vi "CreateLicenseKeyPC.vi"(8 "error in":errorcluster, 10 "Serial number":string, 11 "IP address (localhost)":string="169.254.1.19") -> (0 "error out":errorcluster)   [LabVIEW 2020]
uses:
  <vilib>/Utility/config.llb/Write Key (String).vi
  <vilib>/WebDAVClient/Advanced/Put File.vi
  <vilib>/Utility/config.llb/NI_LVConfig.lvlib
  <vilib>/WebDAVClient/NI_WebDAV.lvlib
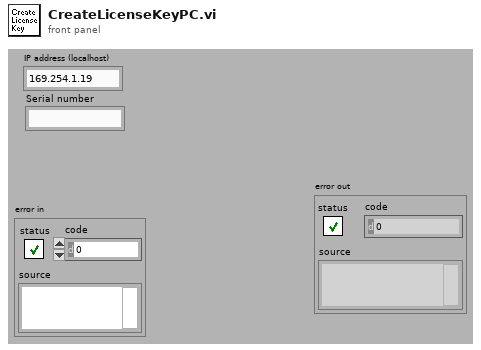
[diagram p1: front panel]
types:
  T1 = typedef "NI_LVConfig.lvlib/Config Data RefNum.ctl" = refnum<k1>
  T2 = typedef "NI_WebDAV.lvlib/SessionHandle.ctl" = refnum<k1>
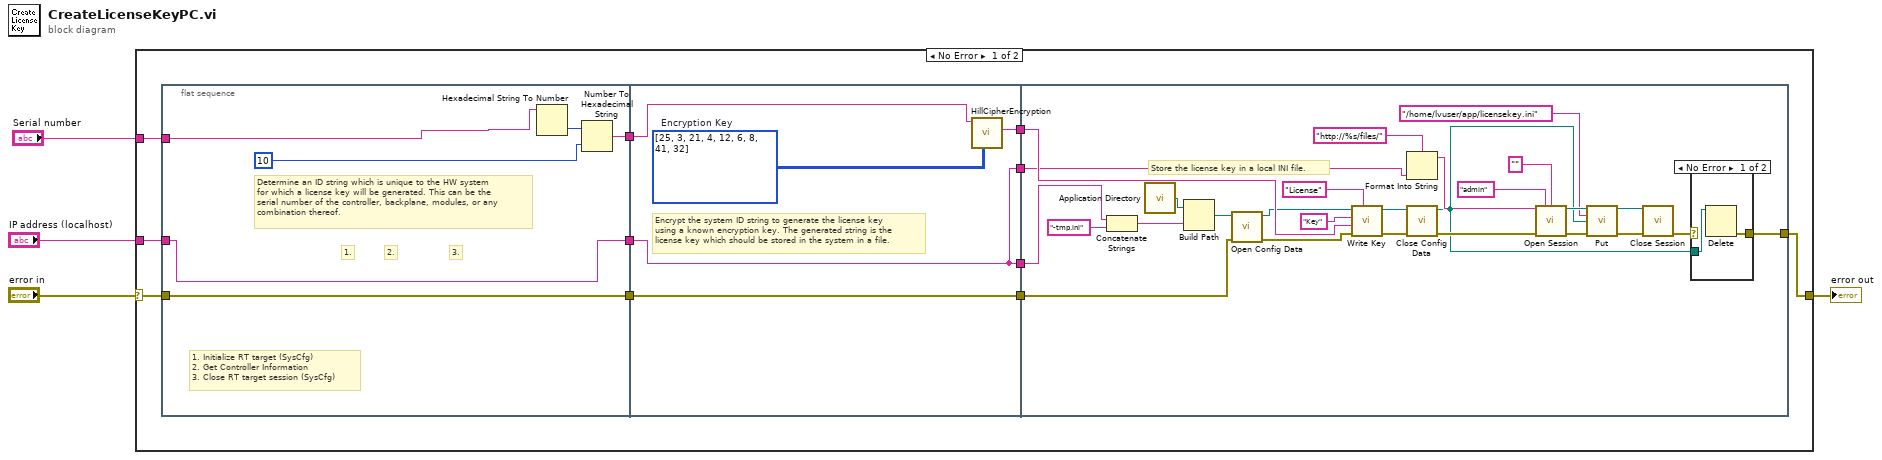
[diagram p0: block diagram]
diagram:
  n1 = case shown="No Error" "error in" {
    selector: "error in" -> [w7 w57]
    tunnel: "IP address (localhost)" -> [w8 _]
    tunnel: [w6 w57] -> w2
    tunnel: "Serial number" -> [w5 _]
    frame No Error {
      n2 = flat-sequence {
        tunnel: [w20] -> w15
        tunnel: [w17] -> w14
        tunnel: w8 -> [w18]
        tunnel: [w18] -> w13
        tunnel: w7 -> [w17]
        tunnel: w5 -> [w16]
        tunnel: w15 -> [w25]
        tunnel: [w24] -> w12
        tunnel: [w23] -> w11
        tunnel: w14 -> [w23]
        tunnel: [w22] -> w10
        tunnel: w13 -> [w22]
        tunnel: [w22] -> w9
        tunnel: w12 -> [w53]
        tunnel: w11 -> [w41]
        tunnel: w10 -> [w46]
        tunnel: w9 -> [w39]
        tunnel: [w28] -> w6
        frame #0 {
          # "3."
          # "2."
          # "1."
          # "1. Initialize RT target (SysCfg)\n2. Get Controller Information\n3. Close RT target session (SysCfg)"
          # "Determine an ID string which is unique to the HW system\nfor which a license key will be generated. This can be the \nserial number of the controller, backplane, modules, or any\ncombination thereof."
          n3 = Hexadecimal String To Number(string=w16) -> (number=w19:u32)  [unwired: 2 in, 1 out]
          n4 = Number To Hexadecimal String(1:i16 10 ("width (-)"), 2:w19) -> (0:w20:string)
        }
        frame #1 {
          w26 = u8[][] [[25, 3, 21], [4, 12, 6], [8, 41, 32]]  # Encryption Key
          # "Encrypt the system ID string to generate the license key\nusing a known encryption key. The generated string is the\nlicense key which should be stored in the system in a file."
          n5 = call "HillCipherEncryption.vi"("Encryption Key"=w26, "Input String"=w25) -> ("Output String (Hex)"=w24:string)  [unwired: 7 in, 2 out]
        }
        frame #2 {
          # "Store the license key in a local INI file."
          n6 = Concatenate Strings(w46, "-tmp.ini" ("string")) -> (w43:string)
          n7 = call <vilib>:"Application Directory.vi"() -> ("Application Directory"=w44:path)
          n8 = Build Path(base path=w44, name or relative path=w43) -> (appended path=w42:path)
          n9 = call <vilib>:"Open Config Data.vi"("error in (no error)"=w41, "configuration file path"=w42) -> ("error out"=w52:errorcluster, "refnum"=w51:T1)  [unwired: 7 in, 1 out]
          n10 = call-poly <vilib>:"Write Key.vi"("section"="License", "error in (no error)"=w52, "value"=w53, "key"="Key", "refnum"=w51) -> ("error out"=w50:errorcluster, "refnum out"=w49:T1)  [unwired: 4 in, 1 out]
          n11 = Format Into String(format string="http://%s/files/", w39) -> (resulting string=w38:string)  [unwired: 2 in, 1 out]
          n12 = call <vilib>:"Close Config Data.vi"("error in (no error)"=w50, "refnum"=w49) -> ("error out"=w35:errorcluster, "file path"=w27:path)  [unwired: 8 in]
          n13 = call <vilib>:"Open Session.vi"("host uri prefix"=w38, "username"="admin", "password"="", "error in (no error)"=w35) -> ("session handle out"=w34:T2, "error out"=w33:errorcluster)  [unwired: 10 in]
          n14 = call-poly <vilib>:"Put.vi"("session handle"=w34, "relative uri"="/home/lvuser/app/licensekey.ini", "local file path"=w27, "error in (no error)"=w33) -> ("session handle out"=w31:T2, "error out"=w30:errorcluster)  [unwired: 9 in, 1 out]
          n15 = call <vilib>:"Close Session.vi"("session handle"=w31, "error in (no error)"=w30) -> ("error out"=w29:errorcluster)  [unwired: 13 in]
          n16 = case shown="No Error" w29 {
            selector: w29 -> [_ w56]
            tunnel: [w55 w56] -> w28
            tunnel: w27 -> [w54 _]
            frame No Error {
              n17 = Delete(path (use dialog)=w54) -> (error out=w55:errorcluster)  [unwired: 4 in, 2 out]
            }
            frame Error {
            }
          }
        }
      }
    }
    frame Error {
    }
  }
  "error out" <- w2
